vi "Remove last frame of waveform with minimal delay on read(1).vi"() -> ()   [LabVIEW 2018]
uses:
  <instrlib>/RIGOL DG4000 Series/Public/Configure/Configure Standard Waveform(Square).vi
  <instrlib>/RIGOL DG4000 Series/Public/Configure/Configure Standard Waveform(Sine).vi
  <vilib>/measure/madcrms.llb/Basic Averaged DC-RMS for 1 Chan.vi
  <instrlib>/RIGOL DS1000 Series/RIGOL DS1000 Series.lvlib
  <instrlib>/RIGOL DG4000 Series/RIGOL DG4000 Series.lvlib
  <vilib>/measure/NI_MAPro.lvlib
panel:
  out "Time taken to complete \nWaveform modification":dbl
  out "Time taken to complete \nScope mesurement":dbl
  out "Time taken to \ncomplete generator":dbl
  out "Time taken to \ncomplete in Seconds":dbl
  in  "Tab Control":enum32{"Sine Wave", "Square Wave"}(tab)
  in  "Frequency (1000 Hz)":dbl=1000.0
  in  "Frequency (1000 Hz) 2":dbl=1000.0
  in  "Duty Cycle (50 %)":dbl=50.0
  out "Waveform Data 2":waveform(dbl)(graph)
  out "RMS value 2":dbl format="%0.2p"
  out "Y min 2":dbl format="%0.2f"
  out "Y max 2":dbl format="%0.2f"
  out "RMS value":dbl format="%0.2p"
  out "Y min":dbl format="%0.2f"
  out "Y max":dbl format="%0.2f"
  in  "VISA Generator":refnum<visa-resource-name>
  in  "Match Frequency to input wave\nfor 2.2 times wave capture":dbl=1000.0
  in  "VISA Scope":refnum<visa-resource-name>
  out "Waveform Data":waveform(dbl)(graph)
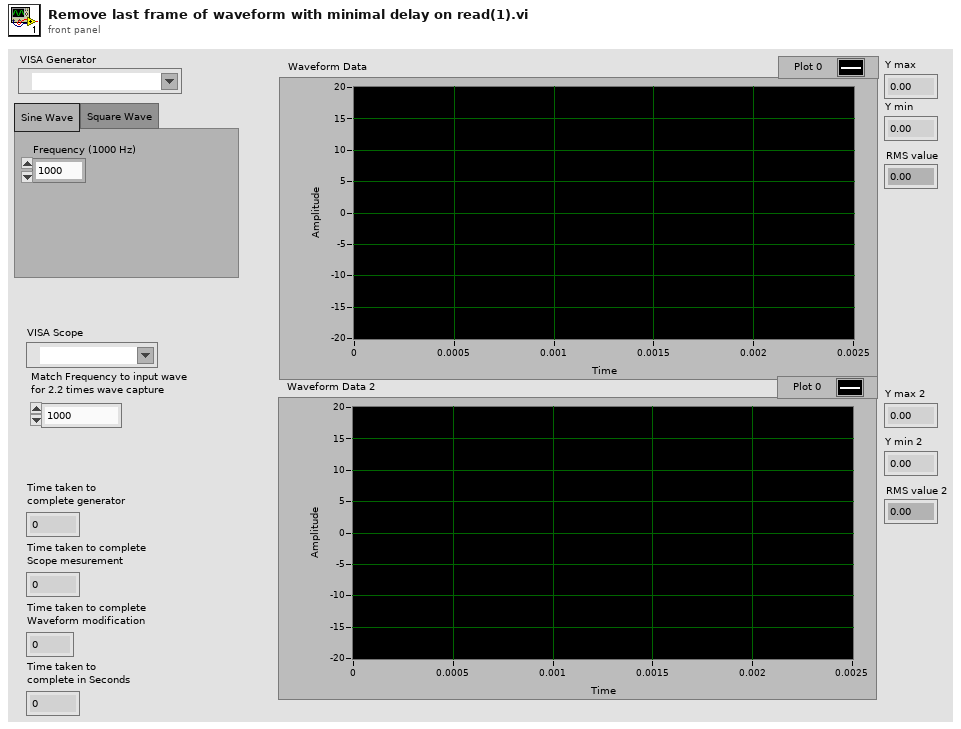
[diagram p1: front panel]
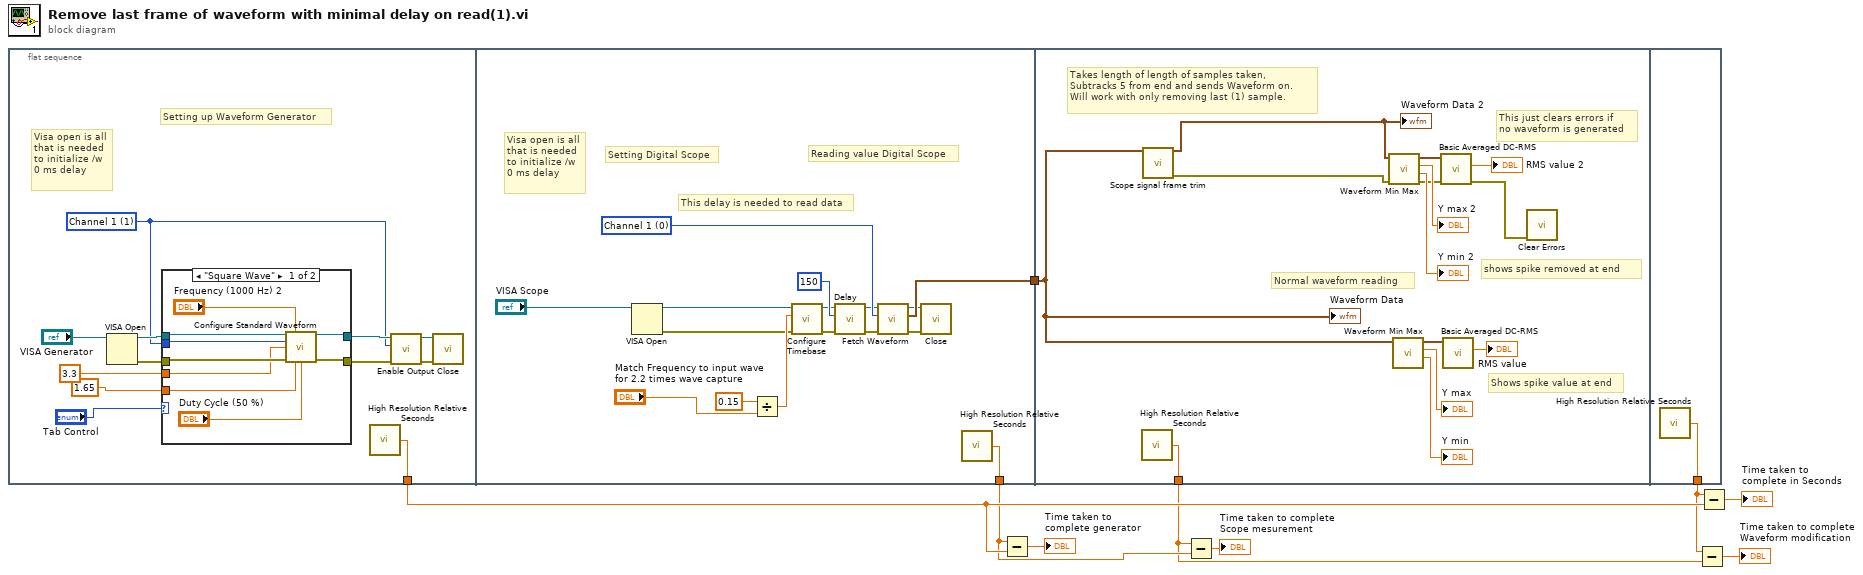
[diagram p0: block diagram]
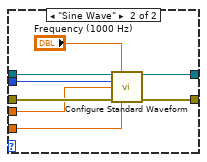
[diagram p2: hidden frame]
diagram:
  n1 = flat-sequence {
    tunnel: [w10] -> w5
    tunnel: [w44] -> w9
    tunnel: [w41] -> w4
    tunnel: w9 -> [w59]
    tunnel: [w55] -> w2
    tunnel: [w69] -> w1
    frame #0 {
      w18 = 1 items=["Channel 1"=1, "Channel 2"=2] ("Output Channel (1: Channel 1)")
      # "Visa open is all\nthat is needed \nto initialize /w\n0 ms delay"
      # "Setting up Waveform Generator"
      n2 = VISA Open(VISA resource name="VISA Generator") -> (VISA resource name=w20:refnum<visa-resource-name>, error out=w14:errorcluster)  [unwired: 4 in]
      n3 = case shown="\"Square Wave\"" "Tab Control" {
        tunnel: w20 -> [w30 w35]
        tunnel: [w29 w36] -> w19
        tunnel: w18 -> [w25 w33]
        tunnel: [w28 w38] -> w15
        tunnel: w14 -> [w27 w37]
        tunnel: 3.3 ("Amplitude (5 Vpp)") -> [w24 w32]
        tunnel: 1.65 ("Offset (0)") -> [w23 w31]
        frame "Square Wave" {
          n4 = call-poly <instrlib>:"Configure Standard Waveform.vi"("VISA resource name"=w30, "Frequency (1000 Hz)"="Frequency (1000 Hz) 2", "Output Channel (1: Channel 1)"=w25, "Amplitude (5 Vpp)"=w24, "error in (no error)"=w27, "Offset (0)"=w23, "Duty Cycle (50 %)"="Duty Cycle (50 %)") -> ("VISA resource name out"=w29:refnum<visa-resource-name>, "error out"=w28:errorcluster)  [unwired: 7 in]
        }
        frame "Sine Wave" {
          n5 = call-poly <instrlib>:"Configure Standard Waveform.vi"("VISA resource name"=w35, "Frequency (1000 Hz)"="Frequency (1000 Hz)", "Output Channel (1: Channel 1)"=w33, "Amplitude (5 Vpp)"=w32, "error in (no error)"=w37, "Offset (0)"=w31) -> ("VISA resource name out"=w36:refnum<visa-resource-name>, "error out"=w38:errorcluster)  [unwired: 8 in]
        }
      }
      n6 = call <vilib>:"High Resolution Relative Seconds.vi"() -> ("relative seconds"=w10:dbl)
      n7 = call <instrlib>:"Enable Output.vi"("error in (no error)"=w15, "Output Channel (1: Channel 1)"=w18, "VISA resource name"=w19) -> ("error out"=w16:errorcluster, "VISA resource name out"=w17:refnum<visa-resource-name>)  [unwired: 7 in]
      n8 = call <instrlib>:"Close.vi"("error in (no error)"=w16, "VISA resource name"=w17) -> ()  [unwired: 9 in, 1 out]
    }
    frame #1 {
      w53 = 0 items=["Channel 1", "Channel 2", "Channel 3", "Channel 4", "EXT", "EXT5", "AC Line", "Digital 0", "Digital 1", "Digital 2", "Digital 3", "Digital 4", "Digital 5", "Digital 6", "Digital 7", "Digital 8", "Digital 9", "Digital 10", "Digital 11", "Digital 12", "Digital 13", "Digital 14", "Digital 15"] ("Trigger Source (0: Channel 1)")
      # "This delay is needed to read data"
      # "Reading value Digital Scope"
      # "Setting Digital Scope"
      # "Visa open is all\nthat is needed \nto initialize /w\n0 ms delay"
      n9 = VISA Open(VISA resource name="VISA Scope") -> (VISA resource name=w43:refnum<visa-resource-name>, error out=w42:errorcluster)  [unwired: 4 in]
      n10 = Divide(x=0.15, y="Match Frequency to input wave\nfor 2.2 times wave capture") -> (x/y=w47:dbl)
      n11 = call <instrlib>:"Configure Timebase.vi"("error in (no error)"=w42, "Timebase (0.0005 s)"=w47, "VISA resource name"=w43) -> ("error out"=w45:errorcluster, "VISA resource name out"=w46:refnum<visa-resource-name>)  [unwired: 7 in]
      n12 = call <instrlib>:"Delay.vi"("error in (no error)"=w45, "Delay (ms)"=u32 150, "VISA resource name"=w46) -> ("error out"=w52:errorcluster, "VISA resource name out"=w40:refnum<visa-resource-name>)  [unwired: 7 in]
      n13 = call <instrlib>:"Fetch Waveform.vi"("error in (no error)"=w52, "Channel (0: Channel 1)"=w53, "VISA resource name"=w40) -> ("error out"=w50:errorcluster, "Waveform Data"=w44:waveform(dbl), "VISA resource name out"=w39:refnum<visa-resource-name>)  [unwired: 6 in]
      n14 = call <instrlib>:"Close.vi"("error in (no error)"=w50, "VISA resource name"=w39) -> ()  [unwired: 9 in, 1 out]
      n15 = call <vilib>:"High Resolution Relative Seconds.vi"() -> ("relative seconds"=w41:dbl)
    }
    frame #2 {
      # "shows spike removed at end"
      # "Shows spike value at end"
      # "This just clears errors if \nno waveform is generated"
      # "Takes length of length of samples taken,\nSubtracks 5 from end and sends Waveform on.\nWill work with only removing last (1) sample."
      # "Normal waveform reading"
      n16 = call <vilib>:"High Resolution Relative Seconds.vi"() -> ("relative seconds"=w55:dbl)
      n17 = call "Scope signal frame trim.vi"("Waveform Data"=w59) -> ("waveform out"=w60:waveform(dbl), "error out"=w56:errorcluster)  [unwired: 13 in]
      "Waveform Data 2" <- w60
      n18 = call <vilib>:"Waveform Min Max.vi"("error in (no error)"=w56, "waveform in"=w60) -> ("error out"=w57:errorcluster, "Y min"=→"Y min 2":dbl, "Y max"=→"Y max 2":dbl, "waveform out"=w62:waveform(dbl))  [unwired: 4 in, 2 out]
      n19 = call <vilib>:"Waveform Min Max.vi"("waveform in"=w59) -> ("Y min"=→"Y min":dbl, "Y max"=→"Y max":dbl, "waveform out"=w66:waveform(dbl))  [unwired: 5 in, 3 out]
      n20 = call-poly <vilib>:"Basic Averaged DC-RMS.vi"("error in (no error)"=w57, "signal in"=w62) -> ("error out"=w58:errorcluster, "RMS value"=→"RMS value 2":dbl)  [unwired: 6 in, 2 out]
      n21 = call-poly <vilib>:"Basic Averaged DC-RMS.vi"("signal in"=w66) -> ("RMS value"=→"RMS value":dbl)  [unwired: 7 in, 3 out]
      n22 = call <vilib>:"Clear Errors.vi"("error in (no error)"=w58) -> ()  [unwired: 5 in, 2 out]
      "Waveform Data" <- w59
    }
    frame #3 {
      n23 = call <vilib>:"High Resolution Relative Seconds.vi"() -> ("relative seconds"=w69:dbl)
    }
  }
  n24 = Subtract(x=w4, y=w5) -> (x-y=→"Time taken to \ncomplete generator":dbl)
  n25 = Subtract(x=w2, y=w4) -> (x-y=→"Time taken to complete \nScope mesurement":dbl)
  n26 = Subtract(x=w1, y=w2) -> (x-y=→"Time taken to complete \nWaveform modification":dbl)
  n27 = Subtract(x=w1, y=w5) -> (x-y=→"Time taken to \ncomplete in Seconds":dbl)
